vi "Wavefrom Values from Cursors.vi"(8 "Error In":errorcluster, 9 "Waveform In":waveform(dbl), 11 "Waveform Graph":refnum<vi>) -> (0 "Error Out":errorcluster, 1 "Waveform Values":waveform(dbl), 2 "Cursor Values":dbl[](array[numeric]))   [LabVIEW 2016]
uses:
  <vilib>/Waveform/WDTOps.llb/WDT Waveform Duration DBL.vi
  <vilib>/Waveform/WDTOps.llb/WDT Get XY Value DBL.vi
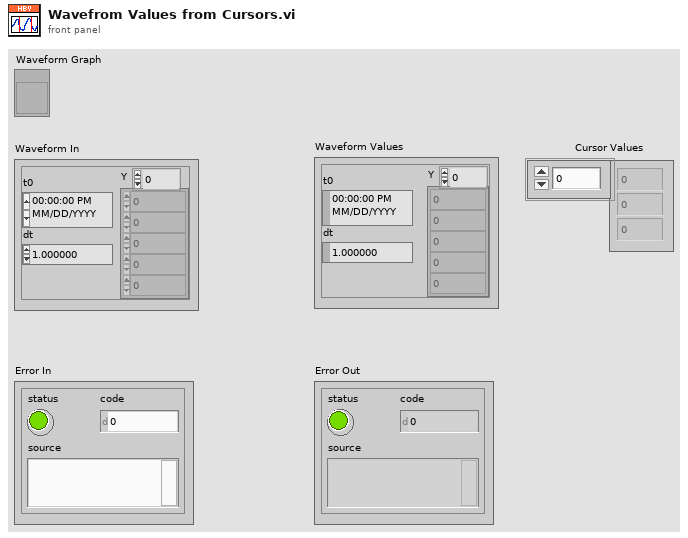
[diagram p1: front panel]
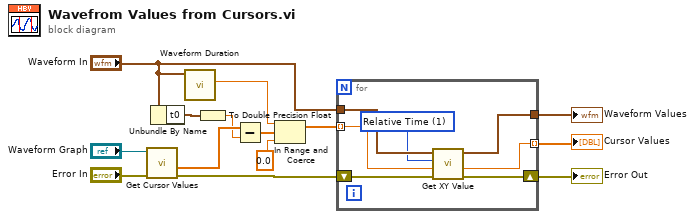
[diagram p0: block diagram]
diagram:
  n1 = call "Get Cursor Values.vi"("error in (no error)"="Error In", "Waveform Graph Ref"="Waveform Graph") -> ("error out"=w4:errorcluster, "Cursor values"=w13:dbl[])  [unwired: 7 in]
  n2 = Unbundle By Name("Waveform In") -> ("t0"=w11:timestamp)
  n3 = call-poly <vilib>:"Waveform Duration.vi"("waveform in"="Waveform In") -> ("duration"=w14:dbl)  [unwired: 8 in, 2 out]
  n4 = To Double Precision Float(number=w11) -> (double precision float=w12:dbl)
  n5 = Subtract(x=w13, y=w12) -> (x-y=w8:dbl[])
  n6 = In Range and Coerce(upper limit=w14, x=w8, lower limit=0.0 ("duration")) -> (coerced(x)=w7:dbl[])  [unwired: 1 out]
  n7 = for {
    tunnel: w7 -> [w21] mode=indexing
    tunnel: "Waveform In" -> [w20]
    shift-right: [w18] -> w5
    shift-left: w4 -> [w17]
    tunnel: [w16] -> w3
    tunnel: [w15] -> w1 mode=indexing
    w19 = u16 1 items=["Samples", "Relative Time"] ("Y position format")
    n8 = call-poly <vilib>:"Get XY Value.vi"("error in (no error)"=w17, "Y position"=w21, "Y position format"=w19, "waveform in"=w20) -> ("error out"=w18:errorcluster, "Y value"=w15:dbl, "waveform out"=w16:waveform(dbl))  [unwired: 3 in, 2 out]
  }
  "Error Out" <- w5
  "Waveform Values" <- w3
  "Cursor Values" <- w1
